vi "FLAGSdll_Test.vi"(8 "error in (no error)":errorcluster) -> (0 "error out":errorcluster, 3 "Passed?":bool)   [LabVIEW 2015]
panel:
  out "kFlag 2":i32
  out "kFlag 3":i32
  out "kFlag":i32
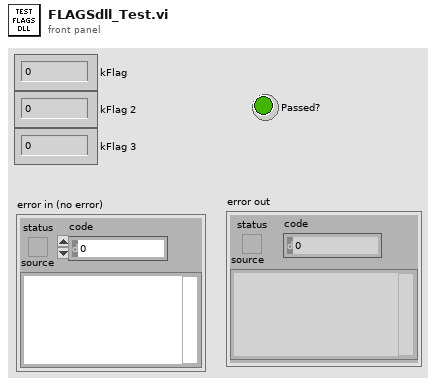
[diagram p1: front panel]
types:
  T1 = cluster{"kFlag":i32, "ierr":i32, "herr":string, "herr length":i32, "hFlag length":i32}
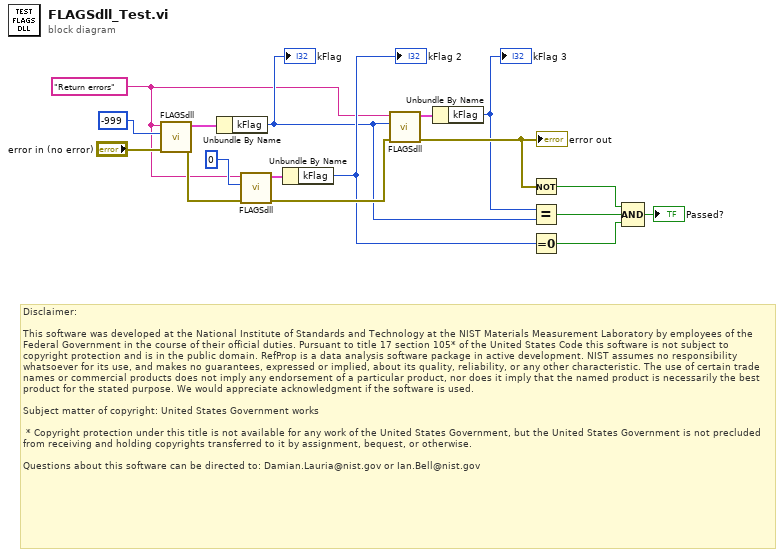
[diagram p0: block diagram]
diagram:
  w1 = "Return errors" ("hFlag")
  # "Disclaimer:\n\nThis software was developed at the National Institute of Standards and Technology at the NIST Materials Measurement Laboratory by employees of the Federal Government in the course of their official duties. Pursuant to title 17 section 105* of the United States Code this software is not subject to copyright protection and is in the public domain. RefProp is a data analysis software package in active development. NIST assumes no responsibility whatsoever for its use, and makes no guarantees, expressed or implied, about its quality, reliability, or any other characteristic. The use of certain trade names or commercial products does not imply any endorsement of a particular product, nor does it imply that the named product is necessarily the best product for the stated purpose. We would appreciate acknowledgment if the software is used.\n \nSubject matter of copyright: United States Government works\n  \n * Copyright protection under this title is not available for any work of the United States Government, but the United States Government is not precluded from receiving and holding copyrights transferred to it by assignment, bequest, or otherwise.\n\nQuestions about this software can be directed to: Damian.Lauria@nist.gov or Ian.Bell@nist.gov"
  n1 = call "FLAGSdll.vi"("error in (no error)"="error in (no error)", "jFlag"=-999, "hFlag"=w1) -> ("error out"=w16:errorcluster, "Outputs"=w7:T1)  [unwired: 7 in]
  n2 = Unbundle By Name(w7) -> ("kFlag"=w4:i32)
  "kFlag" <- w4
  n3 = call "FLAGSdll.vi"("error in (no error)"=w16, "jFlag"=0, "hFlag"=w1) -> ("error out"=w14:errorcluster, "Outputs"=w6:T1)  [unwired: 7 in]
  n4 = Unbundle By Name(w6) -> ("kFlag"=w5:i32)
  "kFlag 2" <- w5
  n5 = call "FLAGSdll.vi"("error in (no error)"=w14, "jFlag"=w4, "hFlag"=w1) -> ("error out"=w12:errorcluster, "Outputs"=w3:T1)  [unwired: 7 in]
  "error out" <- w12
  n6 = Unbundle By Name(w3) -> ("kFlag"=w2:i32)
  "kFlag 3" <- w2
  n7 = Not(x=w12) -> (.not. x?=w11:bool)
  n8 = Equal?(x=w2, y=w4) -> (x = y?=w10:bool)
  n9 = Equal To 0?(x=w5) -> (x = 0?=w9:bool)
  n10 = Compound Arithmetic op=AND(w11, w10, w9) -> (→"Passed?":bool)
